vi "Clear VI.vi"(8 "error in":errorcluster, 11 "VI Refnum In":refnum<vi>) -> (0 "error out":errorcluster, 3 "VI Refnum Out":refnum<vi>)   [LabVIEW 2020]
doc: "Remove all breakpoints and probes from the active VI. The VI is saved but the VI reference is not closed."
uses:
  src/Type Definitions/Class Name--enum.ctl
  <vilib>/Utility/traverseref.llb/TRef TravTarget.ctl
  <vilib>/Utility/miscctls.llb/LVBreakpointStatusEnum.ctl
  <vilib>/Utility/traverseref.llb/VI Scripting - Traverse.lvlib
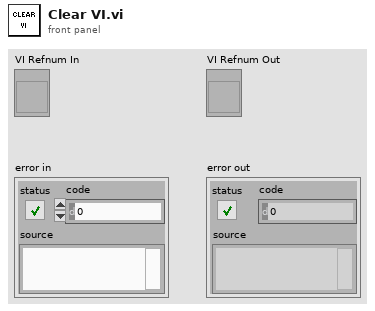
[diagram p1: front panel]
types:
  T1 = typedef "Class Name--enum.ctl" = enum16{"Node", "Wire"}
  T2 = typedef "TRef TravTarget.ctl" = enum16{"FP", "BD", "Other"}
  T3 = typedef "LVBreakpointStatusEnum.ctl" = enum8{"Cleared Break", "Enabled Break", "Disabled Break"}
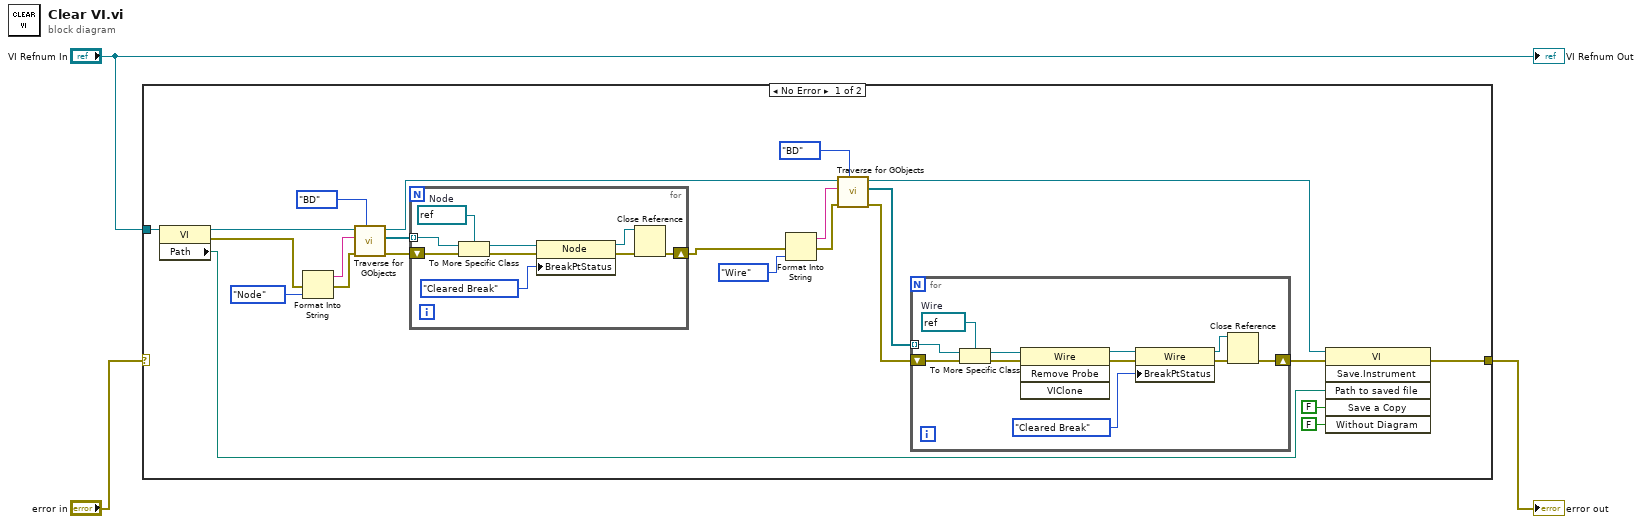
[diagram p0: block diagram]
diagram:
  n1 = case shown="No Error" "error in" {
    selector: "error in" -> [_ w47]
    tunnel: [w4 w47] -> w2
    tunnel: "VI Refnum In" -> [w7 _]
    frame No Error {
      n2 = property class="VI"(reference=w7) -> (reference out=w6:refnum<vi>, error out=w20:errorcluster, "Path"=w5:path)  [unwired: 1 in]
      n3 = Format Into String(error in=w20, Class_Name--enum."Node" ("input 1")) -> (resulting string=w19:string, error out=w26:errorcluster)  [unwired: 2 in]
      n4 = call <vilib>:"Traverse for GObjects.vi"("Traverse Target"=TRef_TravTarget."BD", "error in (no error)"=w26, "Class Name"=w19, "VI Refnum"=w6) -> ("error out"=w25:errorcluster, "References"=w16:refnum<vi>[], "dup VI Refnum"=w12:refnum<vi>)  [unwired: 4 in, 1 out]
      n5 = for {
        tunnel: w16 -> [w42] mode=indexing
        shift-right: [w43] -> w22
        shift-left: w25 -> [w46]
        w41 = refnum<vi> refnum  # Node
        n6 = To More Specific Class(target class=w41, reference=w42, error in=w46) -> (specific class reference=w38:refnum<vi>, error out=w45:errorcluster)
        n7 = property class="Node"(reference=w38, error in=w45, "BreakPtStatus"=LVBreakpointStatusEnum."Cleared Break" ("Breakpoint Status")) -> (reference out=w39:refnum<vi>, error out=w44:errorcluster)
        n8 = Close Reference(reference=w39, error in (no error)=w44) -> (error out=w43:errorcluster)
      }
      n9 = Format Into String(error in=w22, Class_Name--enum."Wire" ("input 1")) -> (resulting string=w15:string, error out=w23:errorcluster)  [unwired: 2 in]
      n10 = call <vilib>:"Traverse for GObjects.vi"("Traverse Target"=TRef_TravTarget."BD", "error in (no error)"=w23, "Class Name"=w15, "VI Refnum"=w12) -> ("error out"=w21:errorcluster, "References"=w11:refnum<vi>[], "dup VI Refnum"=w10:refnum<vi>)  [unwired: 4 in, 1 out]
      n11 = for {
        tunnel: w11 -> [w32] mode=indexing
        shift-right: [w34] -> w24
        shift-left: w21 -> [w37]
        w30 = refnum<vi> refnum  # Wire
        n12 = To More Specific Class(target class=w30, reference=w32, error in=w37) -> (specific class reference=w31:refnum<vi>, error out=w36:errorcluster)
        n13 = invoke class="Wire" method="Remove Probe"(reference=w31, error in=w36) -> (reference out=w29:refnum<vi>, error out=w35:errorcluster)  [unwired: 2 in, 2 out]
        n14 = property class="Wire"(reference=w29, error in=w35, "BreakPtStatus"=LVBreakpointStatusEnum."Cleared Break" ("Breakpoint Status")) -> (reference out=w28:refnum<vi>, error out=w33:errorcluster)
        n15 = Close Reference(reference=w28, error in (no error)=w33) -> (error out=w34:errorcluster)
      }
      n16 = invoke class="VI" method="Save.Instrument"(reference=w10, error in=w24, "Path to saved file"=w5, "Save a Copy"=FALSE, "Without Diagram"=FALSE) -> (error out=w4:errorcluster)  [unwired: 1 in, 5 out]
    }
    frame Error {
      # "Pass error without further action"
    }
  }
  "error out" <- w2
  "VI Refnum Out" <- "VI Refnum In"
